vi "FT10_Unitherm Reconnect.vi"(8 "error in (no error)":errorcluster, 11 "VISA Refnum in":refnum<visa-resource-name>="COM4") -> (0 "error out":errorcluster, 3 "VISA Refnum out":refnum<visa-resource-name>="COM4")   [LabVIEW 2015]
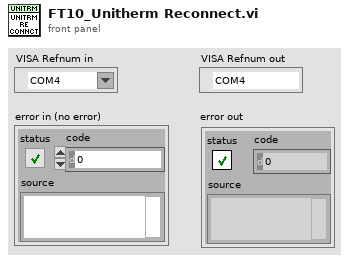
[diagram p1: front panel]
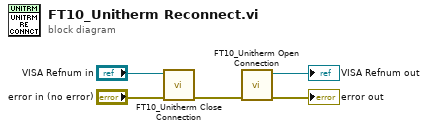
[diagram p0: block diagram]
diagram:
  n1 = call "FT10_Unitherm Close Connection.vi"("error in (no error)"="error in (no error)", "VISA Refnum in"="VISA Refnum in") -> ("error out"=w1:errorcluster)  [unwired: 8 in, 1 out]
  n2 = call "FT10_Unitherm Open Connection.vi"("error in (no error)"=w1) -> ("error out"=→"error out":errorcluster, "VISA Refnum out"=→"VISA Refnum out":refnum<visa-resource-name>)  [unwired: 9 in]
